vi "Create-heartbeat.vi"(8 "error in (no error)":errorcluster, 9 "Sender ID":i32, 10 "Sender":string) -> (0 "error out":errorcluster, 3 "Heartbeat out":refnum<class "Heartbeat.lvclass">)   [LabVIEW 2013, in "Messages.lvlib" / "Heartbeat.lvclass"]
uses:
  Heartbeat.lvclass
  Base-messages.ctl
  Messages.lvlib
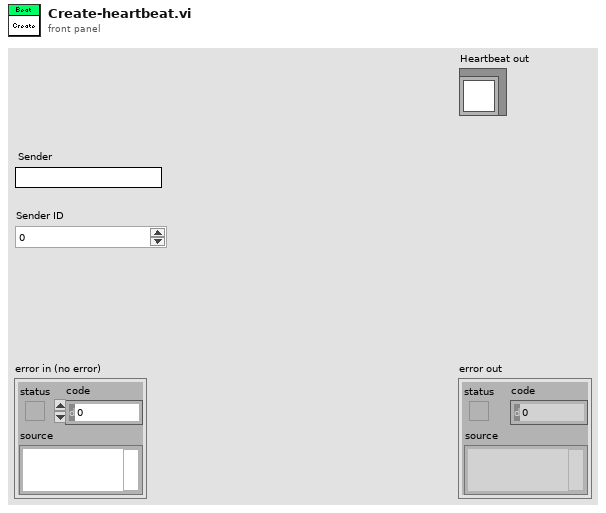
[diagram p1: front panel]
types:
  T1 = typedef "Messages.lvlib/Base-messages.ctl" = enum16{"Heartbeat", "Error", "Start client", "Stop client", "Get clients", "Query status", "Send status", "Action"}
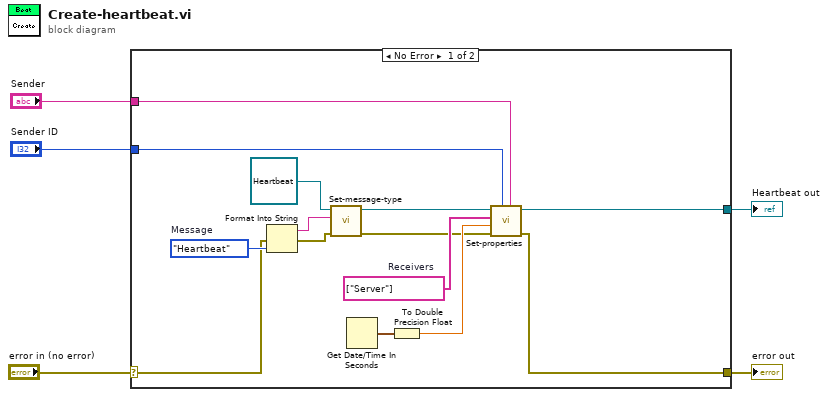
[diagram p0: block diagram]
diagram:
  n1 = case shown="No Error" "error in (no error)" {
    selector: "error in (no error)" -> [w9 w20]
    tunnel: [w8 w20] -> w4
    tunnel: [w7 _] -> w3
    tunnel: "Sender" -> [w15 _]
    tunnel: "Sender ID" -> [w14 _]
    frame No Error {
      w13 = string[] ["Server"]  # Receivers
      w19 = Base-messages."Heartbeat"  # Message
      n2 = Format Into String(error in=w9, w19) -> (resulting string=w18:string, error out=w17:errorcluster)  [unwired: 2 in]
      n3 = call-dynamic "Set-message-type.vi"("error in (no error)"=w17, "Message type"=w18, "Message in"=refnum<class "Heartbeat.lvclass"> refnum) -> ("error out"=w10:errorcluster, "Message out"=w16:refnum<class "Heartbeat.lvclass">)  [unwired: 7 in]
      n4 = Get Date/Time In Seconds() -> (seconds since 1Jan1904=w12:timestamp)
      n5 = To Double Precision Float(number=w12) -> (double precision float=w11:dbl)
      n6 = call-dynamic "Set-properties.vi"("Sender type"=w15, "Sender ID"=w14, "error in (no error)"=w10, "Send time"=w11, "Receivers"=w13, "Message in"=w16) -> ("error out"=w8:errorcluster, "Message out"=w7:refnum<class "Heartbeat.lvclass">)  [unwired: 4 in]
    }
    frame Error {
    }
  }
  "error out" <- w4
  "Heartbeat out" <- w3
